vi "Image2ObjectsDistances.vi"(3 "error in (no error)":errorcluster, 5 "Image Src":T2) -> (0 "error out":errorcluster, 2 "Objects bottom cords":T1(array[cluster]))   [LabVIEW 2009, in "ImageAnalysis.lvlib"]
uses:
  ImageAnalysis.lvlib
  <vilib>/vision/Image Controls.llb/IMAQ Image.ctl
  ImageProcessing.lvlib
  <vilib>/vision/NI_Vision_Development_Module.lvlib
  ControlProject/NetworkVarTarget.lvlib
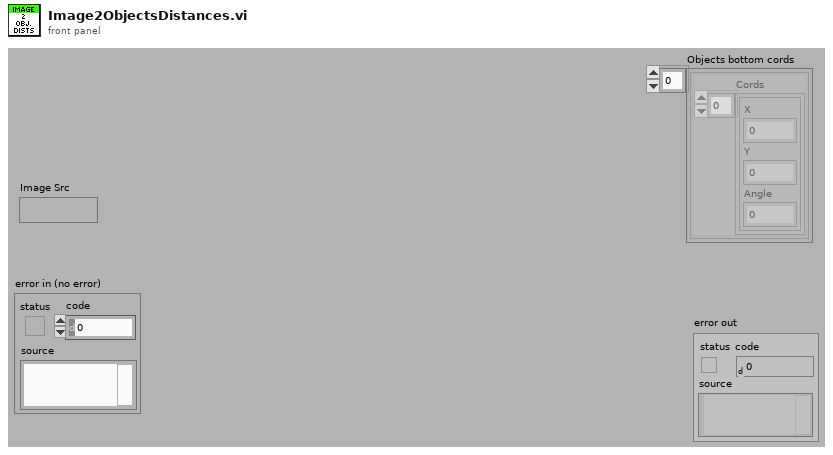
[diagram p1: front panel]
types:
  T1 = cluster{"Cords":cluster{"X":dbl, "Y":dbl, "Angle":dbl}[]}[]
  T2 = typedef "IMAQ Image.ctl" = refnum<image>
  T3 = typedef "Image Type" = u32
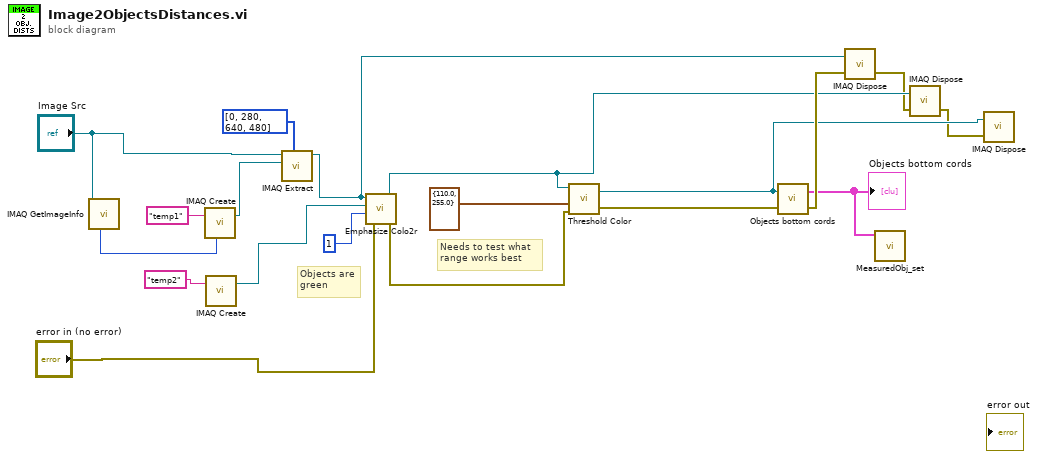
[diagram p0: block diagram]
diagram:
  # "Needs to test what \nrange works best"
  # "Objects are\ngreen"
  n1 = call "IMAQ GetImageInfo"("Image"="Image Src") -> ("Image Type"=w9:T3)  [unwired: 3 in, 7 out]
  n2 = call "IMAQ Create"("Image Name"="temp1", "Image Type"=w9) -> ("New Image"=w11:T2)  [unwired: 3 in, 1 out]
  n3 = call "IMAQ Create"("Image Name"="temp2") -> ("New Image"=w13:T2)  [unwired: 4 in, 1 out]
  n4 = call "IMAQ Extract"("Optional Rectangle"=i32[] [0, 280, 640, 480], "Image Dst"=w11, "Image Src"="Image Src") -> ("Image Dst Out"=w7:T2)  [unwired: 7 in, 1 out]
  n5 = call "Emphasize Colo2r.vi"("error in (no error)"="error in (no error)", "Color"=i8 1, "Image Dst"=w13, "Image Src"=w7) -> ("error out"=w18:errorcluster, "Image Out"=w5:T2)
  n6 = call "Threshold Color.vi"("error in (no error)"=w18, "Range"=cluster{"Lower value":sgl, "Upper value":sgl} {"Lower value"=110.0, "Upper value"=255.0}, "Image Src"=w5) -> ("error out"=w15:errorcluster, "Image Dst Out"=w3:T2)  [unwired: 1 in]
  n7 = call "Objects bottom cords.vi"("error in (no error)"=w15, "Image"=w3) -> ("error out"=w6:errorcluster, "Objects bottom cords"=w1:T1)
  "Objects bottom cords" <- w1
  n8 = call "IMAQ Dispose"("Image"=w7, "error in (no error)"=w6) -> ("error out"=w4:errorcluster)  [unwired: 4 in]
  n9 = call "MeasuredObj_set.vi"("MeasuredObjects"=w1) -> ()  [unwired: 10 in, 1 out]
  n10 = call "IMAQ Dispose"("Image"=w5, "error in (no error)"=w4) -> ("error out"=w2:errorcluster)  [unwired: 4 in]
  n11 = call "IMAQ Dispose"("Image"=w3, "error in (no error)"=w2) -> ()  [unwired: 4 in, 1 out]
